vi "testbufferrollover.vi"() -> ()   [LabVIEW 2017]
uses:
  <vilib>/addons/InsightCM/Devices/Shared/Common/DVRBuffer/controls/DVRElement.ctl
  <vilib>/addons/InsightCM/Devices/Shared/Common/DVRBuffer/DVRBuffer.lvlib
panel:
  out "Array 2":T1[](array[typedef])
  out "Array":T1[](array[typedef])
  out "replaced dvr":u32
  out "logical AND":bool
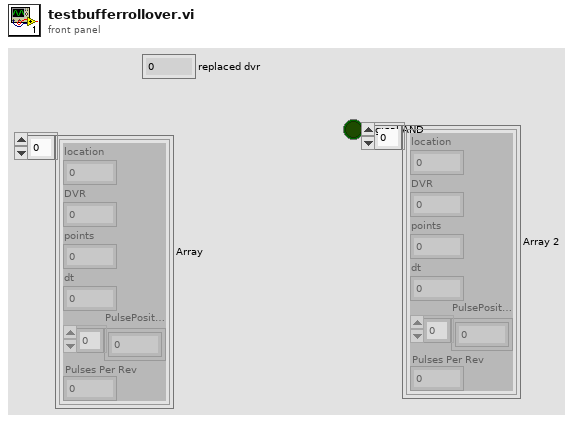
[diagram p1: front panel]
types:
  T1 = typedef "DVRBuffer.lvlib/DVRElement.ctl" = cluster{"location":u32, "DVR":u32, "points":i32, "dt":dbl, "PulsePositions":dbl[], "Pulses Per Rev":dbl}
  T2 = cluster{"location":bool, "DVR":bool, "points":bool, "dt":bool, "PulsePositions":bool[], "Pulses Per Rev":bool}[]
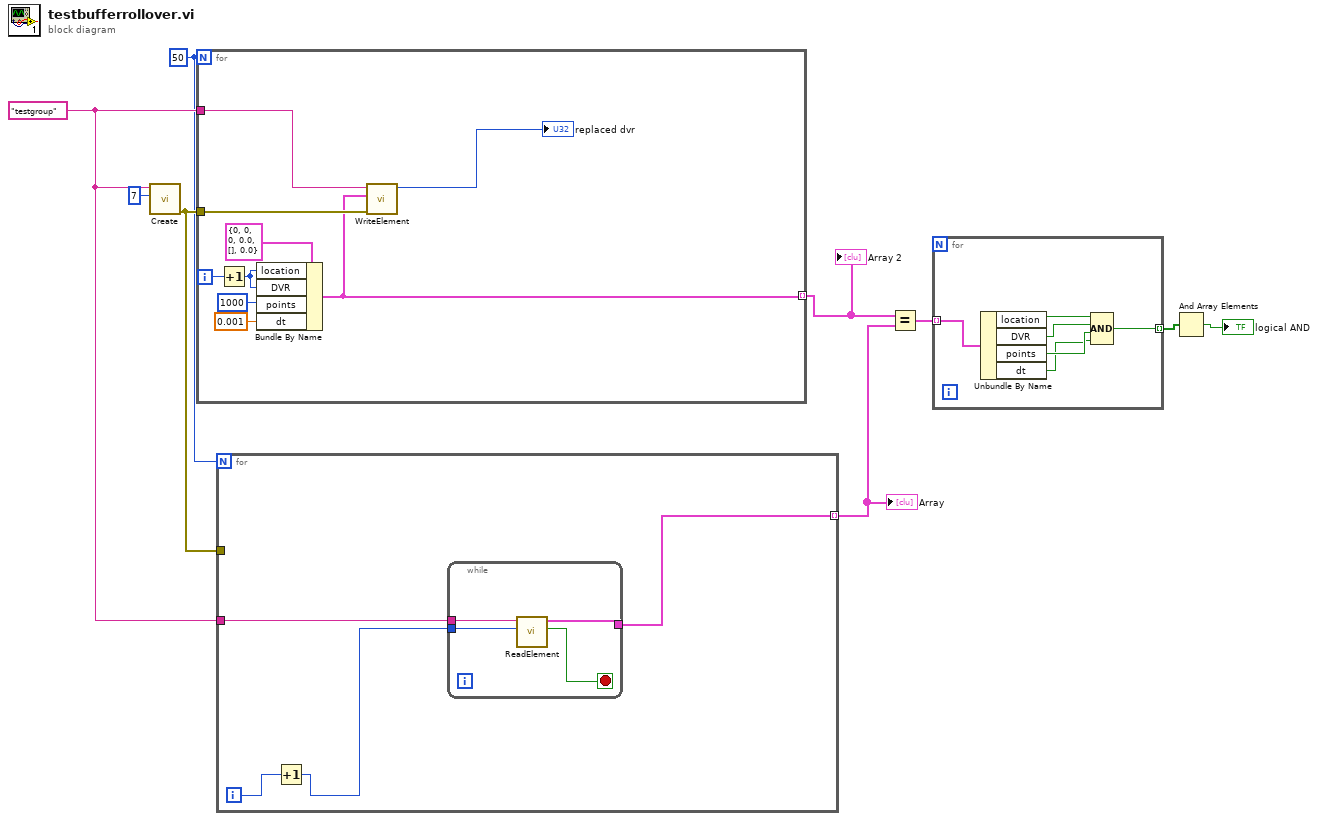
[diagram p0: block diagram]
diagram:
  w1 = 50
  w7 = "testgroup" ("name")
  n1 = call <vilib>:"Create.vi"("size"=7, "name"=w7) -> ("error out"=w8:errorcluster)  [unwired: 8 in, 1 out]
  n2 = for {
    N: w1 -> [_]
    tunnel: w7 -> [w18]
    tunnel: w8 -> [w16]
    tunnel: [w13] -> w5 mode=indexing
    i -> [w11]
    n3 = Increment(x=w11) -> (x+1=w10:i32)
    n4 = Bundle By Name(cluster=T1 {"location"=0, "DVR"=0, "points"=0, "dt"=0.0, "PulsePositions"=[], "Pulses Per Rev"=0.0} ("dvr element"), "location"=w10, "DVR"=w10, "points"=1000, "dt"=0.001) -> (w13:T1)
    n5 = call <vilib>:"WriteElement.vi"("error in (no error)"=w16, "dvr element"=w13, "name"=w18) -> ("replaced dvr"=→"replaced dvr":u32)  [unwired: 6 in, 2 out]
  }
  "Array 2" <- w5
  n6 = for {
    N: w1 -> [_]
    tunnel: w8 -> [_]
    tunnel: w7 -> [w22]
    tunnel: [w21] -> w6 mode=indexing
    i -> [w20]
    n7 = Increment(x=w20) -> (x+1=w19:i32)
    n8 = while {
      tunnel: w19 -> [w26]
      tunnel: w22 -> [w25]
      tunnel: [w24] -> w21
      stop <- w23 stop-if-true
      n9 = call <vilib>:"ReadElement.vi"("buffer location"=w26, "name"=w25) -> ("found"=w23:bool, "DVR element"=w24:T1)  [unwired: 7 in, 1 out]
    }
  }
  "Array" <- w6
  n10 = Equal?(x=w5, y=w6) -> (x = y?=w4:T2)
  n11 = for {
    tunnel: w4 -> [w32] mode=indexing
    tunnel: [w27] -> w3 mode=indexing
    n12 = Unbundle By Name(w32) -> ("location"=w31:bool, "DVR"=w30:bool, "points"=w29:bool, "dt"=w28:bool)
    n13 = Compound Arithmetic op=AND(w31, w30, w29, w28) -> (w27:bool)
  }
  n14 = And Array Elements(Boolean array=w3) -> (logical AND=→"logical AND":bool)
